vi "Visa Address Check and fix.vi"(0 "Instruments":T1[](array[typedef]), 1 "NML Addresses":string[](array[string]), 2 "Name":string, 3 "Address":u16(ring) items=["GPIB 0 - Address 11", "GPIB 0 - Address 14"]) -> (4 "Array":variant[](array[variant]), 5 "Firmware":string, 6 "Wait Time (mS)":u32, 7 "VISA resource name":refnum<visa-resource-name>, 8 "Title":string, 9 "NML Addresses":string[](array[string]), 10 "Model":string)   [LabVIEW 2025]
doc: "Author: Scott Hannahs <sth@magnet.fsu.edu>\n\nThis software is licensed for use under the “MIT License\"\nCopyright (c) 2025 Scott Hannahs, sth@sth@magnet.sthnet.net\n\nPermission is hereby granted, free of charge, to any person obtaining a copy of this software and associated documentation files (the \"Software\"), to deal in the Software without restriction, including without limitation the rights to use, copy, modify, merge, publish, distribute, sublicense, and/or sell copies of the Software, and to permit persons to whom the Software is furnished to do so, subject to the following conditions: The above copyright notice and this permission notice shall be included in all copies or substantial portions of the Software.\n\nTHE SOFTWARE IS PROVIDED \"AS IS\", WITHOUT WARRANTY OF ANY KIND, EXPRESS OR IMPLIED, INCLUDING BUT NOT LIMITED TO THE WARRANTIES OF MERCHANTABILITY, FITNESS FOR A PARTICULAR PURPOSE AND NONINFRINGEMENT. IN NO EVENT SHALL THE AUTHORS OR COPYRIGHT HOLDERS BE LIABLE FOR ANY CLAIM, DAMAGES OR OTHER LIABILITY, WHETHER IN AN ACTION OF CONTRACT, TORT OR OTHERWISE, ARISING FROM, OUT OF OR IN CONNECTION WITH THE SOFTWARE OR THE USE OR OTHER DEALINGS IN THE SOFTWARE."
uses:
  Sub Controls/Instrument Match.ctl
  SetupGlobals.vi
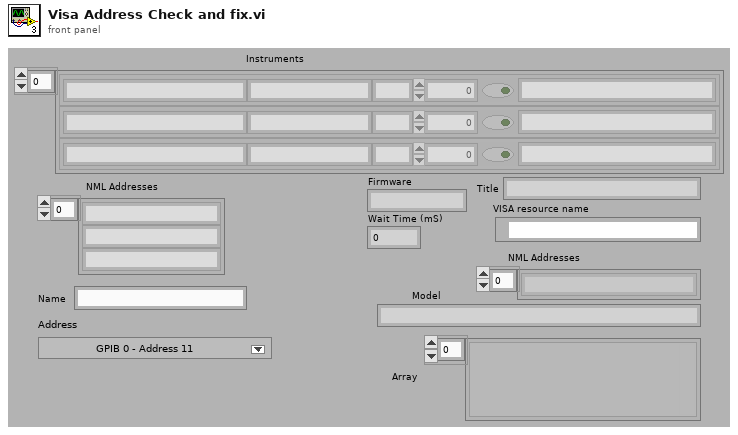
[diagram p1: front panel]
types:
  T1 = typedef "Instrument Match.ctl" = cluster{"Model":string, "Manufacturer":string, "Term Character":string, "Wait Time (mS)":u32, "Wait for SRQ":bool, "Type":string}
  T2 = typedef "Instrument IDN.ctl" = cluster{"VISA Address":string, "Status":u16, "Manufacturer":string, "Model":string, "Info":string, "Info 2":string, "Misc Data":variant}
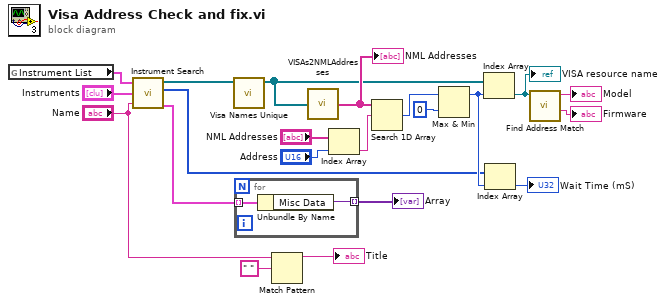
[diagram p0: block diagram]
diagram:
  n1 = global read "SetupGlobals.vi" "Instrument List"() -> (w5:T2[])
  n2 = call "Instrument Search.vi"("Instrument List"=w5, "Instruments"="Instruments", "Name"="Name") -> ("VISA resource names"=w9:refnum<visa-resource-name>[], "Wait Times (mS)"=w2:u32[], "Instrument Array"=w4:T2[])  [unwired: 1 in]
  n3 = call "Visa Names Unique.vi"("VISA resource names In"=w9) -> ("Unique VISA resource namesOut"=w10:refnum<visa-resource-name>[])  [unwired: 10 in]
  n4 = for {
    tunnel: w4 -> [w23] mode=indexing
    tunnel: [w22] -> w7 mode=indexing
    n5 = Unbundle By Name(w23) -> ("Misc Data"=w22:variant)
  }
  "Array" <- w7
  n6 = Match Pattern(string="Name", regular expression=" ") -> (before substring=→"Title":string)  [unwired: 1 in, 3 out]
  n7 = call "VISAs2NMLAddresses.vi"("VISA Resource Names"=w10) -> ("NML Addresses"=w16:string[])
  "NML Addresses" <- w16
  n8 = Index Array(array="NML Addresses", index="Address") -> (element=w17:string)
  n9 = Search 1D Array(1D array=w16, element=w17) -> (index of element=w15:i32)  [unwired: 1 in]
  n10 = Max & Min(x=w15, y=0) -> (max(x,y)=w3:i32)  [unwired: 1 out]
  n11 = Index Array(array=w10, index=w3) -> (element=w8:refnum<visa-resource-name>)
  "VISA resource name" <- w8
  n12 = Index Array(array=w2, index=w3) -> (element=→"Wait Time (mS)":u32)
  n13 = call "Find Address Match.vi"("VISA resource name"=w8) -> ("Firmware"=→"Firmware":string, "Model"=→"Model":string)  [unwired: 3 in, 2 out]
